vi "main(Test DQMH modules).vi"() -> ()   [LabVIEW 2018, in "Application.lvlib"] (continued)
        n1265 = Build Array("Apps.UI Update", "MEAS.AllRelaysOFF2", "Apps.WaitForEvent") -> (w2918:string[])
        n1266 = for {
          tunnel: [w2978] -> w2924 mode=indexing
          shift-right: [w2979] -> w2925
          shift-left: w2920 -> [w2977]
          tunnel: w2918 -> [w2976] mode=indexing
          n1267 = call "App enquece.vi"("Priority Enquece"=TRUE, "command"=w2976, "queue in"=w2977) -> ("error out"=w2978:errorcluster, "Queue out"=w2979:refnum<queue>)  [unwired: 7 in]
        }
        n1268 = call "FGV DRV stand.vi"() -> ("Sub-Test.DCV"=w2910:bool)  [unwired: 10 in, 1 out]
        n1269 = case shown="True" w2910 {
          tunnel: [w2965 w2975] -> w2926
          frame False {
            n1270 = Build Array("WaitFor", "MEAS.requestAC") -> (w2965:string[])
          }
          frame True {
            n1271 = Build Array("Test DRV 37", "Test DRV 38", "Test DRV 39", "Test DRV 40", "Test DRV 41", "Test DRV 42", "MEAS.requestAC") -> (w2975:string[])
          }
        }
        n1272 = Merge Errors(w2924) -> (w2917:errorcluster)
        n1273 = Reverse 1D Array(array=w2926) -> (reversed array=w2927:string[])
        n1274 = for {
          tunnel: w2927 -> [w2985] mode=indexing
          tunnel: [w2984] -> w2923 mode=indexing
          shift-right: [w2983] -> w2916
          shift-left: w2925 -> [w2986]
          tunnel: w2917 -> [w2982]
          n1275 = call "App enquece.vi"("Priority Enquece"=TRUE, "error in (no error)"=w2982, "command"=w2985, "queue in"=w2986) -> ("error out"=w2984:errorcluster, "Queue out"=w2983:refnum<queue>)  [unwired: 6 in]
        }
        n1276 = call "FGV DRV stand.vi"() -> ("Sub-Test.DCV"=w2909:bool)  [unwired: 10 in, 1 out]
        n1277 = Merge Errors(w2923) -> (w2922:errorcluster)
        n1278 = case shown="False" w2909 {
          tunnel: [w2938 w2954] -> w2921
          frame True {
            w2939 = T9 {"command"="", "data"=variant} ("element")
            n1279 = Initialize Array(TRUE, 6 ("dimension size")) -> (w2942:bool[])
            n1280 = To Variant(anything=T3."mux10_1_channel7" ("mux10_1(x6)_encode")) -> (Variant=w2951:variant)
            n1281 = To Variant(anything=T4."demux1_10_channel7" ("demux1_10(x6)_encode")) -> (Variant=w2947:variant)
            n1282 = To Variant(anything=w2942) -> (Variant=w2941:variant)
            n1283 = Bundle By Name(cluster=w2939, "command"="MEAS.mux10-1", "data"=w2951) -> (w2946:T9)
            n1284 = Bundle By Name(cluster=w2939, "command"="MEAS.demux1-10", "data"=w2947) -> (w2945:T9)
            n1285 = Bundle By Name(cluster=w2939, "command"="MEAS.eMIC", "data"=w2941) -> (w2940:T9)
            n1286 = Build Array(w2946, w2945, w2940) -> (w2938:T9[])
          }
          frame False {
            w2955 = T9 {"command"="", "data"=variant} ("element")
            n1287 = Initialize Array(TRUE, 6 ("dimension size")) -> (w2958:bool[])
            n1288 = To Variant(anything=T4."demux1_10_channel7" ("demux1_10(x6)_encode")) -> (Variant=w2962:variant)
            n1289 = To Variant(anything=w2958) -> (Variant=w2957:variant)
            n1290 = Bundle By Name(cluster=w2955, "command"="MEAS.demux1-10", "data"=w2962) -> (w2961:T9)
            n1291 = Bundle By Name(cluster=w2955, "command"="MEAS.eMIC", "data"=w2957) -> (w2956:T9)
            n1292 = Build Array(w2961, w2956) -> (w2954:T9[])
          }
        }
        n1293 = Reverse 1D Array(array=w2921) -> (reversed array=w2915:T9[])
        n1294 = for {
          tunnel: w2915 -> [w2997] mode=indexing
          tunnel: [w2994] -> w2928 mode=indexing
          tunnel: w2922 -> [w2993]
          tunnel: w2916 -> [w2991]
          n1295 = Unbundle By Name(w2997) -> ("command"=w2996:string, "data"=w2995:variant)
          n1296 = call "App enquece.vi"("Priority Enquece"=TRUE, "error in (no error)"=w2993, "command data"=w2995, "command"=w2996, "queue in"=w2991) -> ("error out"=w2994:errorcluster)  [unwired: 5 in, 1 out]
        }
        n1297 = Merge Errors(w2931, w2928) -> (w2932:errorcluster)
      }
      frame "Test Channel 8" {
        w2999 = T9 {"command"="", "data"=variant} ("element")
        w3037 = 8  # DUT channel (1-10)
        n1298 = disable-structure shown="LOGGING==TRUE" {
          disable-tunnel: w3032 -> [w3063 _]
          frame condition #0 (active) {
            n1299 = Empty String/Path?(string/path=w3063) -> (empty?=w3065:bool)
            n1300 = Select(t="Quece timeout", s=w3065, f=w3063) -> (s? t:f=w3062:string)
            n1301 = call "string log (SubVI).vi"("state Name"=w3062) -> ()  [unwired: 9 in, 2 out]
          }
          frame condition #1 {
          }
        }
        n1302 = Build Array("Apps.UI Update", "MEAS.AllRelaysOFF2", "Apps.WaitForEvent") -> (w3019:string[])
        n1303 = for {
          tunnel: [w3053] -> w3026 mode=indexing
          shift-right: [w3054] -> w3028
          shift-left: w3021 -> [w3052]
          tunnel: w3019 -> [w3051] mode=indexing
          n1304 = call "App enquece.vi"("Priority Enquece"=TRUE, "command"=w3051, "queue in"=w3052) -> ("error out"=w3053:errorcluster, "Queue out"=w3054:refnum<queue>)  [unwired: 7 in]
        }
        n1305 = call "FGV DRV stand.vi"() -> ("Sub-Test.DCV"=w3013:bool)  [unwired: 10 in, 1 out]
        n1306 = case shown="True" w3013 {
          tunnel: [w3040 w3050] -> w3029
          frame False {
            n1307 = Build Array("WaitFor", "MEAS.requestAC") -> (w3040:string[])
          }
          frame True {
            n1308 = Build Array("Test DRV 43", "Test DRV 44", "Test DRV 45", "Test DRV 46", "Test DRV 47", "Test DRV 48", "MEAS.requestAC") -> (w3050:string[])
          }
        }
        n1309 = Merge Errors(w3026) -> (w3018:errorcluster)
        n1310 = Reverse 1D Array(array=w3029) -> (reversed array=w3030:string[])
        n1311 = for {
          tunnel: w3030 -> [w3060] mode=indexing
          tunnel: [w3059] -> w3025 mode=indexing
          shift-right: [w3058] -> w3027
          shift-left: w3028 -> [w3061]
          tunnel: w3018 -> [w3057]
          n1312 = call "App enquece.vi"("Priority Enquece"=TRUE, "error in (no error)"=w3057, "command"=w3060, "queue in"=w3061) -> ("error out"=w3059:errorcluster, "Queue out"=w3058:refnum<queue>)  [unwired: 6 in]
        }
        n1313 = Merge Errors(w3025) -> (w3024:errorcluster)
        n1314 = Initialize Array(TRUE, 6 ("dimension size")) -> (w3002:bool[])
        n1315 = To Variant(anything=T3."mux10_1_channel8" ("mux10_1(x6)_encode")) -> (Variant=w3011:variant)
        n1316 = To Variant(anything=T4."demux1_10_channel8" ("demux1_10(x6)_encode")) -> (Variant=w3007:variant)
        n1317 = To Variant(anything=w3002) -> (Variant=w3001:variant)
        n1318 = Bundle By Name(cluster=w2999, "command"="MEAS.mux10-1", "data"=w3011) -> (w3006:T9)
        n1319 = Bundle By Name(cluster=w2999, "command"="MEAS.demux1-10", "data"=w3007) -> (w3005:T9)
        n1320 = Bundle By Name(cluster=w2999, "command"="MEAS.eMIC", "data"=w3001) -> (w3000:T9)
        n1321 = Build Array(w3006, w3005, w3000) -> (w3023:T9[])
        n1322 = Reverse 1D Array(array=w3023) -> (reversed array=w3022:T9[])
        n1323 = for {
          tunnel: w3022 -> [w3071] mode=indexing
          tunnel: [w3068] -> w3031 mode=indexing
          tunnel: w3024 -> [w3067]
          tunnel: w3027 -> [w3072]
          n1324 = Unbundle By Name(w3071) -> ("command"=w3070:string, "data"=w3069:variant)
          n1325 = call "App enquece.vi"("Priority Enquece"=TRUE, "error in (no error)"=w3067, "command data"=w3069, "command"=w3070, "queue in"=w3072) -> ("error out"=w3068:errorcluster)  [unwired: 5 in, 1 out]
        }
        n1326 = Merge Errors(w3034, w3031) -> (w3035:errorcluster)
      }
      frame "Test Channel 9" {
        w3074 = T9 {"command"="", "data"=variant} ("element")
        w3113 = 9  # DUT channel (1-10)
        n1327 = disable-structure shown="LOGGING==TRUE" {
          disable-tunnel: w3108 -> [w3138 _]
          frame condition #0 (active) {
            n1328 = Empty String/Path?(string/path=w3138) -> (empty?=w3140:bool)
            n1329 = Select(t="Quece timeout", s=w3140, f=w3138) -> (s? t:f=w3137:string)
            n1330 = call "string log (SubVI).vi"("state Name"=w3137) -> ()  [unwired: 9 in, 2 out]
          }
          frame condition #1 {
          }
        }
        n1331 = Build Array("Apps.UI Update", "MEAS.AllRelaysOFF2", "Apps.WaitForEvent") -> (w3094:string[])
        n1332 = for {
          tunnel: [w3128] -> w3102 mode=indexing
          shift-right: [w3129] -> w3104
          shift-left: w3097 -> [w3127]
          tunnel: w3094 -> [w3126] mode=indexing
          n1333 = call "App enquece.vi"("Priority Enquece"=TRUE, "command"=w3126, "queue in"=w3127) -> ("error out"=w3128:errorcluster, "Queue out"=w3129:refnum<queue>)  [unwired: 7 in]
        }
        n1334 = call "FGV DRV stand.vi"() -> ("Sub-Test.DCV"=w3088:bool)  [unwired: 10 in, 1 out]
        n1335 = Merge Errors(w3102) -> (w3093:errorcluster)
        n1336 = case shown="True" w3088 {
          tunnel: [w3115 w3125] -> w3105
          frame False {
            n1337 = Build Array("WaitFor", "MEAS.requestAC") -> (w3115:string[])
          }
          frame True {
            n1338 = Build Array("Test DRV 49", "Test DRV 50", "Test DRV 51", "Test DRV 52", "Test DRV 53", "Test DRV 54", "MEAS.requestAC") -> (w3125:string[])
          }
        }
        n1339 = Reverse 1D Array(array=w3105) -> (reversed array=w3106:string[])
        n1340 = for {
          tunnel: w3106 -> [w3135] mode=indexing
          tunnel: [w3134] -> w3101 mode=indexing
          shift-right: [w3133] -> w3103
          shift-left: w3104 -> [w3136]
          tunnel: w3093 -> [w3132]
          n1341 = call "App enquece.vi"("Priority Enquece"=TRUE, "error in (no error)"=w3132, "command"=w3135, "queue in"=w3136) -> ("error out"=w3134:errorcluster, "Queue out"=w3133:refnum<queue>)  [unwired: 6 in]
        }
        n1342 = Merge Errors(w3101) -> (w3100:errorcluster)
        n1343 = Initialize Array(TRUE, 6 ("dimension size")) -> (w3077:bool[])
        n1344 = To Variant(anything=T3."mux10_1_channel9" ("mux10_1(x6)_encode")) -> (Variant=w3086:variant)
        n1345 = To Variant(anything=T4."demux1_10_channel9" ("demux1_10(x6)_encode")) -> (Variant=w3082:variant)
        n1346 = To Variant(anything=w3077) -> (Variant=w3076:variant)
        n1347 = Bundle By Name(cluster=w3074, "command"="MEAS.mux10-1", "data"=w3086) -> (w3081:T9)
        n1348 = Bundle By Name(cluster=w3074, "command"="MEAS.demux1-10", "data"=w3082) -> (w3080:T9)
        n1349 = Bundle By Name(cluster=w3074, "command"="MEAS.eMIC", "data"=w3076) -> (w3075:T9)
        n1350 = Build Array(w3081, w3080, w3075) -> (w3099:T9[])
        n1351 = Reverse 1D Array(array=w3099) -> (reversed array=w3098:T9[])
        n1352 = for {
          tunnel: w3098 -> [w3146] mode=indexing
          tunnel: [w3143] -> w3107 mode=indexing
          tunnel: w3100 -> [w3142]
          tunnel: w3103 -> [w3147]
          n1353 = Unbundle By Name(w3146) -> ("command"=w3145:string, "data"=w3144:variant)
          n1354 = call "App enquece.vi"("Priority Enquece"=TRUE, "error in (no error)"=w3142, "command data"=w3144, "command"=w3145, "queue in"=w3147) -> ("error out"=w3143:errorcluster)  [unwired: 5 in, 1 out]
        }
        n1355 = Merge Errors(w3110, w3107) -> (w3111:errorcluster)
      }
      frame "Test Channel 10" {
        w3150 = T9 {"command"="", "data"=variant} ("element")
        w3187 = 10  # DUT channel (1-10)
        n1356 = disable-structure shown="LOGGING==TRUE" {
          disable-tunnel: w3183 -> [w3213 _]
          frame condition #0 (active) {
            n1357 = Empty String/Path?(string/path=w3213) -> (empty?=w3215:bool)
            n1358 = Select(t="Quece timeout", s=w3215, f=w3213) -> (s? t:f=w3212:string)
            n1359 = call "string log (SubVI).vi"("state Name"=w3212) -> ()  [unwired: 9 in, 2 out]
          }
          frame condition #1 {
          }
        }
        n1360 = Build Array("Apps.UI Update", "MEAS.AllRelaysOFF2", "Apps.WaitForEvent") -> (w3170:string[])
        n1361 = for {
          tunnel: [w3203] -> w3177 mode=indexing
          shift-right: [w3204] -> w3179
          shift-left: w3172 -> [w3202]
          tunnel: w3170 -> [w3201] mode=indexing
          n1362 = call "App enquece.vi"("Priority Enquece"=TRUE, "command"=w3201, "queue in"=w3202) -> ("error out"=w3203:errorcluster, "Queue out"=w3204:refnum<queue>)  [unwired: 7 in]
        }
        n1363 = call "FGV DRV stand.vi"() -> ("Sub-Test.DCV"=w3164:bool)  [unwired: 10 in, 1 out]
        n1364 = case shown="True" w3164 {
          tunnel: [w3190 w3200] -> w3180
          frame False {
            n1365 = Build Array("WaitFor", "MEAS.requestAC") -> (w3190:string[])
          }
          frame True {
            n1366 = Build Array("Test DRV 55", "Test DRV 56", "Test DRV 57", "Test DRV 58", "Test DRV 59", "Test DRV 60", "MEAS.requestAC") -> (w3200:string[])
          }
        }
        n1367 = Merge Errors(w3177) -> (w3169:errorcluster)
        n1368 = Reverse 1D Array(array=w3180) -> (reversed array=w3181:string[])
        n1369 = for {
          tunnel: w3181 -> [w3210] mode=indexing
          tunnel: [w3209] -> w3176 mode=indexing
          shift-right: [w3208] -> w3178
          shift-left: w3179 -> [w3211]
          tunnel: w3169 -> [w3207]
          n1370 = call "App enquece.vi"("Priority Enquece"=TRUE, "error in (no error)"=w3207, "command"=w3210, "queue in"=w3211) -> ("error out"=w3209:errorcluster, "Queue out"=w3208:refnum<queue>)  [unwired: 6 in]
        }
        n1371 = Merge Errors(w3176) -> (w3175:errorcluster)
        n1372 = Initialize Array(TRUE, 6 ("dimension size")) -> (w3148:bool[])
        n1373 = To Variant(anything=T3."mux10_1_channel10" ("mux10_1(x6)_encode")) -> (Variant=w3161:variant)
        n1374 = To Variant(anything=T4."demux1_10_channel10" ("demux1_10(x6)_encode")) -> (Variant=w3157:variant)
        n1375 = To Variant(anything=w3148) -> (Variant=w3153:variant)
        n1376 = Bundle By Name(cluster=w3150, "command"="MEAS.mux10-1", "data"=w3161) -> (w3156:T9)
        n1377 = Bundle By Name(cluster=w3150, "command"="MEAS.demux1-10", "data"=w3157) -> (w3155:T9)
        n1378 = Bundle By Name(cluster=w3150, "command"="MEAS.eMIC", "data"=w3153) -> (w3152:T9)
        n1379 = Build Array(w3156, w3155, w3152) -> (w3174:T9[])
        n1380 = Reverse 1D Array(array=w3174) -> (reversed array=w3173:T9[])
        n1381 = for {
          tunnel: w3173 -> [w3221] mode=indexing
          tunnel: [w3218] -> w3182 mode=indexing
          tunnel: w3175 -> [w3217]
          tunnel: w3178 -> [w3222]
          n1382 = Unbundle By Name(w3221) -> ("command"=w3220:string, "data"=w3219:variant)
          n1383 = call "App enquece.vi"("Priority Enquece"=TRUE, "error in (no error)"=w3217, "command data"=w3219, "command"=w3220, "queue in"=w3222) -> ("error out"=w3218:errorcluster)  [unwired: 5 in, 1 out]
        }
        n1384 = Merge Errors(w3185, w3182) -> (w3163:errorcluster)
      }
      frame "Test Channel 10A" {
        w3229 = T9 {"command"="", "data"=variant} ("element")
        w3250 = T9 {"command"="", "data"=variant} ("element")
        w3271 = 10  # DUT channel (1-10)
        n1385 = disable-structure shown="LOGGING==TRUE" {
          disable-tunnel: w3266 -> [w3295 _]
          frame condition #0 (active) {
            n1386 = Empty String/Path?(string/path=w3295) -> (empty?=w3297:bool)
            n1387 = Select(t="Quece timeout", s=w3297, f=w3295) -> (s? t:f=w3294:string)
            n1388 = call "string log (SubVI).vi"("state Name"=w3294) -> ()  [unwired: 9 in, 2 out]
          }
          frame condition #1 {
          }
        }
        n1389 = Bundle By Name(cluster=w3250, "command"="Apps.UI Update", "data"="A") -> (w3249:T9)
        n1390 = Bundle By Name(cluster=w3250, "command"="MEAS.AllRelaysOFF2") -> (w3248:T9)
        n1391 = Bundle By Name(cluster=w3250, "command"="Apps.WaitForEvent") -> (w3247:T9)
        n1392 = Build Array(w3249, w3248, w3247) -> (w3255:T9[])
        n1393 = call "FGV DRV stand.vi"() -> ("Sub-Test.DCV"=w3243:bool)  [unwired: 10 in, 1 out]
        n1394 = for {
          tunnel: [w3285] -> w3261 mode=indexing
          shift-right: [w3286] -> w3263
          shift-left: w3256 -> [w3284]
          tunnel: w3255 -> [w3283] mode=indexing
          n1395 = Unbundle By Name(w3283) -> ("command"=w3282:string, "data"=w3281:variant)
          n1396 = call "App enquece.vi"("Priority Enquece"=TRUE, "command data"=w3281, "command"=w3282, "queue in"=w3284) -> ("error out"=w3285:errorcluster, "Queue out"=w3286:refnum<queue>)  [unwired: 6 in]
        }
        n1397 = case shown="True" w3243 {
          tunnel: [w3274 w3280] -> w3264
          frame False {
            n1398 = Build Array("WaitFor", "MEAS.requestAC") -> (w3274:string[])
          }
          frame True {
            n1399 = Build Array("Test DRV 55", "WaitForA", "MEAS.requestAC") -> (w3280:string[])
          }
        }
        n1400 = Merge Errors(w3261) -> (w3254:errorcluster)
        n1401 = Reverse 1D Array(array=w3264) -> (reversed array=w3242:string[])
        n1402 = for {
          tunnel: w3242 -> [w3292] mode=indexing
          tunnel: [w3291] -> w3260 mode=indexing
          shift-right: [w3290] -> w3262
          shift-left: w3263 -> [w3293]
          tunnel: w3254 -> [w3289]
          n1403 = call "App enquece.vi"("Priority Enquece"=TRUE, "error in (no error)"=w3289, "command"=w3292, "queue in"=w3293) -> ("error out"=w3291:errorcluster, "Queue out"=w3290:refnum<queue>)  [unwired: 6 in]
        }
        n1404 = Merge Errors(w3260) -> (w3259:errorcluster)
        n1405 = Initialize Array(FALSE ("element"), 6 ("dimension size")) -> (w3225:bool[])
        n1406 = Initialize Array(TRUE, 1 ("dimension size")) -> (w3224:bool[])
        n1407 = Replace Array Subset(array=w3225, new element=w3224) -> (w3223:bool[])  [unwired: 1 in]
        n1408 = To Variant(anything=T3."mux10_1_channel10" ("mux10_1(x6)_encode")) -> (Variant=w3240:variant)
        n1409 = To Variant(anything=T4."demux1_10_channel10" ("demux1_10(x6)_encode")) -> (Variant=w3236:variant)
        n1410 = To Variant(anything=w3223) -> (Variant=w3232:variant)
        n1411 = Bundle By Name(cluster=w3229, "command"="MEAS.mux10-1", "data"=w3240) -> (w3235:T9)
        n1412 = Bundle By Name(cluster=w3229, "command"="MEAS.demux1-10", "data"=w3236) -> (w3234:T9)
        n1413 = Bundle By Name(cluster=w3229, "command"="MEAS.eMIC", "data"=w3232) -> (w3231:T9)
        n1414 = Build Array(w3235, w3234, w3231) -> (w3258:T9[])
        n1415 = Reverse 1D Array(array=w3258) -> (reversed array=w3257:T9[])
        n1416 = for {
          tunnel: w3257 -> [w3303] mode=indexing
          tunnel: [w3300] -> w3265 mode=indexing
          tunnel: w3259 -> [w3299]
          tunnel: w3262 -> [w3304]
          n1417 = Unbundle By Name(w3303) -> ("command"=w3302:string, "data"=w3301:variant)
          n1418 = call "App enquece.vi"("Priority Enquece"=TRUE, "error in (no error)"=w3299, "command data"=w3301, "command"=w3302, "queue in"=w3304) -> ("error out"=w3300:errorcluster)  [unwired: 5 in, 1 out]
        }
        n1419 = Merge Errors(w3268, w3265) -> (w3269:errorcluster)
      }
      frame "Test Channel 1A" {
        w3311 = T9 {"command"="", "data"=variant} ("element")
        w3332 = T9 {"command"="", "data"=variant} ("element")
        w3353 = 1  # DUT channel (1-10)
        n1420 = disable-structure shown="LOGGING==TRUE" {
          disable-tunnel: w3348 -> [w3377 _]
          frame condition #0 (active) {
            n1421 = Empty String/Path?(string/path=w3377) -> (empty?=w3379:bool)
            n1422 = Select(t="Quece timeout", s=w3379, f=w3377) -> (s? t:f=w3376:string)
            n1423 = call "string log (SubVI).vi"("state Name"=w3376) -> ()  [unwired: 9 in, 2 out]
          }
          frame condition #1 {
          }
        }
        n1424 = Bundle By Name(cluster=w3332, "command"="Apps.UI Update", "data"="A") -> (w3331:T9)
        n1425 = Bundle By Name(cluster=w3332, "command"="MEAS.AllRelaysOFF2") -> (w3330:T9)
        n1426 = Bundle By Name(cluster=w3332, "command"="Apps.WaitForEvent") -> (w3329:T9)
        n1427 = Build Array(w3331, w3330, w3329) -> (w3337:T9[])
        n1428 = for {
          tunnel: [w3367] -> w3343 mode=indexing
          shift-right: [w3368] -> w3345
          shift-left: w3338 -> [w3366]
          tunnel: w3337 -> [w3365] mode=indexing
          n1429 = Unbundle By Name(w3365) -> ("command"=w3364:string, "data"=w3363:variant)
          n1430 = call "App enquece.vi"("Priority Enquece"=TRUE, "command data"=w3363, "command"=w3364, "queue in"=w3366) -> ("error out"=w3367:errorcluster, "Queue out"=w3368:refnum<queue>)  [unwired: 6 in]
        }
        n1431 = call "FGV DRV stand.vi"() -> ("Sub-Test.DCV"=w3325:bool)  [unwired: 10 in, 1 out]
        n1432 = case shown="True" w3325 {
          tunnel: [w3356 w3362] -> w3346
          frame False {
            n1433 = Build Array("WaitFor", "MEAS.requestAC") -> (w3356:string[])
          }
          frame True {
            n1434 = Build Array("Test DRV 1", "WaitForA", "MEAS.requestAC") -> (w3362:string[])
          }
        }
        n1435 = Merge Errors(w3343) -> (w3336:errorcluster)
        n1436 = Reverse 1D Array(array=w3346) -> (reversed array=w3324:string[])
        n1437 = for {
          tunnel: w3324 -> [w3374] mode=indexing
          tunnel: [w3373] -> w3342 mode=indexing
          shift-right: [w3372] -> w3344
          shift-left: w3345 -> [w3375]
          tunnel: w3336 -> [w3371]
          n1438 = call "App enquece.vi"("Priority Enquece"=TRUE, "error in (no error)"=w3371, "command"=w3374, "queue in"=w3375) -> ("error out"=w3373:errorcluster, "Queue out"=w3372:refnum<queue>)  [unwired: 6 in]
        }
        n1439 = Merge Errors(w3342) -> (w3341:errorcluster)
        n1440 = Initialize Array(FALSE ("element"), 6 ("dimension size")) -> (w3307:bool[])
        n1441 = Initialize Array(TRUE, 1 ("dimension size")) -> (w3306:bool[])
        n1442 = Replace Array Subset(array=w3307, new element=w3306) -> (w3305:bool[])  [unwired: 1 in]
        n1443 = To Variant(anything=T3."mux10_1_channel1" ("mux10_1(x6)_encode")) -> (Variant=w3322:variant)
        n1444 = To Variant(anything=T4."demux1_10_channel1" ("demux1_10(x6)_encode")) -> (Variant=w3318:variant)
        n1445 = To Variant(anything=w3305) -> (Variant=w3314:variant)
        n1446 = Bundle By Name(cluster=w3311, "command"="MEAS.mux10-1", "data"=w3322) -> (w3317:T9)
        n1447 = Bundle By Name(cluster=w3311, "command"="MEAS.demux1-10", "data"=w3318) -> (w3316:T9)
        n1448 = Bundle By Name(cluster=w3311, "command"="MEAS.eMIC", "data"=w3314) -> (w3313:T9)
        n1449 = Build Array(w3317, w3316, w3313) -> (w3340:T9[])
        n1450 = Reverse 1D Array(array=w3340) -> (reversed array=w3339:T9[])
        n1451 = for {
          tunnel: w3339 -> [w3385] mode=indexing
          tunnel: [w3382] -> w3347 mode=indexing
          tunnel: w3341 -> [w3381]
          tunnel: w3344 -> [w3386]
          n1452 = Unbundle By Name(w3385) -> ("command"=w3384:string, "data"=w3383:variant)
          n1453 = call "App enquece.vi"("Priority Enquece"=TRUE, "error in (no error)"=w3381, "command data"=w3383, "command"=w3384, "queue in"=w3386) -> ("error out"=w3382:errorcluster)  [unwired: 5 in, 1 out]
        }
        n1454 = Merge Errors(w3350, w3347) -> (w3351:errorcluster)
      }
      frame "Test Channel 2A" {
        w3393 = T9 {"command"="", "data"=variant} ("element")
        w3414 = T9 {"command"="", "data"=variant} ("element")
        w3435 = 2  # DUT channel (1-10)
        n1455 = disable-structure shown="LOGGING==TRUE" {
          disable-tunnel: w3430 -> [w3459 _]
          frame condition #0 (active) {
            n1456 = Empty String/Path?(string/path=w3459) -> (empty?=w3461:bool)
            n1457 = Select(t="Quece timeout", s=w3461, f=w3459) -> (s? t:f=w3458:string)
            n1458 = call "string log (SubVI).vi"("state Name"=w3458) -> ()  [unwired: 9 in, 2 out]
          }
          frame condition #1 {
          }
        }
        n1459 = Bundle By Name(cluster=w3414, "command"="Apps.UI Update", "data"="A") -> (w3413:T9)
        n1460 = Bundle By Name(cluster=w3414, "command"="MEAS.AllRelaysOFF2") -> (w3412:T9)
        n1461 = Bundle By Name(cluster=w3414, "command"="Apps.WaitForEvent") -> (w3411:T9)
        n1462 = Build Array(w3413, w3412, w3411) -> (w3419:T9[])
        n1463 = for {
          tunnel: [w3449] -> w3425 mode=indexing
          shift-right: [w3450] -> w3427
          shift-left: w3420 -> [w3448]
          tunnel: w3419 -> [w3447] mode=indexing
          n1464 = Unbundle By Name(w3447) -> ("command"=w3446:string, "data"=w3445:variant)
          n1465 = call "App enquece.vi"("Priority Enquece"=TRUE, "command data"=w3445, "command"=w3446, "queue in"=w3448) -> ("error out"=w3449:errorcluster, "Queue out"=w3450:refnum<queue>)  [unwired: 6 in]
        }
        n1466 = call "FGV DRV stand.vi"() -> ("Sub-Test.DCV"=w3407:bool)  [unwired: 10 in, 1 out]
        n1467 = case shown="True" w3407 {
          tunnel: [w3438 w3444] -> w3428
          frame False {
            n1468 = Build Array("WaitFor", "MEAS.requestAC") -> (w3438:string[])
          }
          frame True {
            n1469 = Build Array("Test DRV 7", "WaitForA", "MEAS.requestAC") -> (w3444:string[])
          }
        }
        n1470 = Merge Errors(w3425) -> (w3418:errorcluster)
        n1471 = Reverse 1D Array(array=w3428) -> (reversed array=w3406:string[])
        n1472 = for {
          tunnel: w3406 -> [w3456] mode=indexing
          tunnel: [w3455] -> w3424 mode=indexing
          shift-right: [w3454] -> w3426
          shift-left: w3427 -> [w3457]
          tunnel: w3418 -> [w3453]
          n1473 = call "App enquece.vi"("Priority Enquece"=TRUE, "error in (no error)"=w3453, "command"=w3456, "queue in"=w3457) -> ("error out"=w3455:errorcluster, "Queue out"=w3454:refnum<queue>)  [unwired: 6 in]
        }
        n1474 = Initialize Array(FALSE ("element"), 6 ("dimension size")) -> (w3389:bool[])
        n1475 = Merge Errors(w3424) -> (w3423:errorcluster)
        n1476 = Initialize Array(TRUE, 1 ("dimension size")) -> (w3388:bool[])
        n1477 = Replace Array Subset(array=w3389, new element=w3388) -> (w3387:bool[])  [unwired: 1 in]
        n1478 = To Variant(anything=T3."mux10_1_channel2" ("mux10_1(x6)_encode")) -> (Variant=w3404:variant)
        n1479 = To Variant(anything=T4."demux1_10_channel2" ("demux1_10(x6)_encode")) -> (Variant=w3400:variant)
        n1480 = To Variant(anything=w3387) -> (Variant=w3396:variant)
        n1481 = Bundle By Name(cluster=w3393, "command"="MEAS.mux10-1", "data"=w3404) -> (w3399:T9)
        n1482 = Bundle By Name(cluster=w3393, "command"="MEAS.demux1-10", "data"=w3400) -> (w3398:T9)
        n1483 = Bundle By Name(cluster=w3393, "command"="MEAS.eMIC", "data"=w3396) -> (w3395:T9)
        n1484 = Build Array(w3399, w3398, w3395) -> (w3422:T9[])
        n1485 = Reverse 1D Array(array=w3422) -> (reversed array=w3421:T9[])
        n1486 = for {
          tunnel: w3421 -> [w3467] mode=indexing
          tunnel: [w3464] -> w3429 mode=indexing
          tunnel: w3423 -> [w3463]
          tunnel: w3426 -> [w3468]
          n1487 = Unbundle By Name(w3467) -> ("command"=w3466:string, "data"=w3465:variant)
          n1488 = call "App enquece.vi"("Priority Enquece"=TRUE, "error in (no error)"=w3463, "command data"=w3465, "command"=w3466, "queue in"=w3468) -> ("error out"=w3464:errorcluster)  [unwired: 5 in, 1 out]
        }
        n1489 = Merge Errors(w3432, w3429) -> (w3433:errorcluster)
      }
      frame "Test Channel 3A" {
        w3475 = T9 {"command"="", "data"=variant} ("element")
        w3496 = T9 {"command"="", "data"=variant} ("element")
        w3517 = 3  # DUT channel (1-10)
        n1490 = disable-structure shown="LOGGING==TRUE" {
          disable-tunnel: w3512 -> [w3541 _]
          frame condition #0 (active) {
            n1491 = Empty String/Path?(string/path=w3541) -> (empty?=w3543:bool)
            n1492 = Select(t="Quece timeout", s=w3543, f=w3541) -> (s? t:f=w3540:string)
            n1493 = call "string log (SubVI).vi"("state Name"=w3540) -> ()  [unwired: 9 in, 2 out]
          }
          frame condition #1 {
          }
        }
        n1494 = Bundle By Name(cluster=w3496, "command"="Apps.UI Update", "data"="A") -> (w3495:T9)
        n1495 = Bundle By Name(cluster=w3496, "command"="MEAS.AllRelaysOFF2") -> (w3494:T9)
        n1496 = Bundle By Name(cluster=w3496, "command"="Apps.WaitForEvent") -> (w3493:T9)
        n1497 = Build Array(w3495, w3494, w3493) -> (w3501:T9[])
        n1498 = for {
          tunnel: [w3531] -> w3507 mode=indexing
          shift-right: [w3532] -> w3509
          shift-left: w3502 -> [w3530]
          tunnel: w3501 -> [w3529] mode=indexing
          n1499 = Unbundle By Name(w3529) -> ("command"=w3528:string, "data"=w3527:variant)
          n1500 = call "App enquece.vi"("Priority Enquece"=TRUE, "command data"=w3527, "command"=w3528, "queue in"=w3530) -> ("error out"=w3531:errorcluster, "Queue out"=w3532:refnum<queue>)  [unwired: 6 in]
        }
        n1501 = call "FGV DRV stand.vi"() -> ("Sub-Test.DCV"=w3489:bool)  [unwired: 10 in, 1 out]
        n1502 = case shown="True" w3489 {
          tunnel: [w3520 w3526] -> w3510
          frame False {
            n1503 = Build Array("WaitFor", "MEAS.requestAC") -> (w3520:string[])
          }
          frame True {
            n1504 = Build Array("Test DRV 13", "WaitForA", "MEAS.requestAC") -> (w3526:string[])
          }
        }
        n1505 = Merge Errors(w3507) -> (w3500:errorcluster)
        n1506 = Reverse 1D Array(array=w3510) -> (reversed array=w3488:string[])
        n1507 = for {
          tunnel: w3488 -> [w3538] mode=indexing
          tunnel: [w3537] -> w3506 mode=indexing
          shift-right: [w3536] -> w3508
          shift-left: w3509 -> [w3539]
          tunnel: w3500 -> [w3535]
          n1508 = call "App enquece.vi"("Priority Enquece"=TRUE, "error in (no error)"=w3535, "command"=w3538, "queue in"=w3539) -> ("error out"=w3537:errorcluster, "Queue out"=w3536:refnum<queue>)  [unwired: 6 in]
        }
        n1509 = Initialize Array(FALSE ("element"), 6 ("dimension size")) -> (w3471:bool[])
        n1510 = Initialize Array(TRUE, 1 ("dimension size")) -> (w3470:bool[])
        n1511 = Merge Errors(w3506) -> (w3505:errorcluster)
        n1512 = Replace Array Subset(array=w3471, new element=w3470) -> (w3469:bool[])  [unwired: 1 in]
        n1513 = To Variant(anything=T3."mux10_1_channel3" ("mux10_1(x6)_encode")) -> (Variant=w3486:variant)
        n1514 = To Variant(anything=T4."demux1_10_channel3" ("demux1_10(x6)_encode")) -> (Variant=w3482:variant)
        n1515 = To Variant(anything=w3469) -> (Variant=w3478:variant)
        n1516 = Bundle By Name(cluster=w3475, "command"="MEAS.mux10-1", "data"=w3486) -> (w3481:T9)
        n1517 = Bundle By Name(cluster=w3475, "command"="MEAS.demux1-10", "data"=w3482) -> (w3480:T9)
        n1518 = Bundle By Name(cluster=w3475, "command"="MEAS.eMIC", "data"=w3478) -> (w3477:T9)
        n1519 = Build Array(w3481, w3480, w3477) -> (w3504:T9[])
        n1520 = Reverse 1D Array(array=w3504) -> (reversed array=w3503:T9[])
        n1521 = for {
          tunnel: w3503 -> [w3549] mode=indexing
          tunnel: [w3546] -> w3511 mode=indexing
          tunnel: w3505 -> [w3545]
          tunnel: w3508 -> [w3550]
          n1522 = Unbundle By Name(w3549) -> ("command"=w3548:string, "data"=w3547:variant)
          n1523 = call "App enquece.vi"("Priority Enquece"=TRUE, "error in (no error)"=w3545, "command data"=w3547, "command"=w3548, "queue in"=w3550) -> ("error out"=w3546:errorcluster)  [unwired: 5 in, 1 out]
        }
        n1524 = Merge Errors(w3514, w3511) -> (w3515:errorcluster)
      }
      frame "Test Channel 4A" {
        w3557 = T9 {"command"="", "data"=variant} ("element")
        w3578 = T9 {"command"="", "data"=variant} ("element")
        w3599 = 4  # DUT channel (1-10)
        n1525 = disable-structure shown="LOGGING==TRUE" {
          disable-tunnel: w3594 -> [w3623 _]
          frame condition #0 (active) {
            n1526 = Empty String/Path?(string/path=w3623) -> (empty?=w3625:bool)
            n1527 = Select(t="Quece timeout", s=w3625, f=w3623) -> (s? t:f=w3622:string)
            n1528 = call "string log (SubVI).vi"("state Name"=w3622) -> ()  [unwired: 9 in, 2 out]
          }
          frame condition #1 {
          }
        }
        n1529 = Bundle By Name(cluster=w3578, "command"="Apps.UI Update", "data"="A") -> (w3577:T9)
        n1530 = Bundle By Name(cluster=w3578, "command"="MEAS.AllRelaysOFF2") -> (w3576:T9)
        n1531 = Bundle By Name(cluster=w3578, "command"="Apps.WaitForEvent") -> (w3575:T9)
        n1532 = Build Array(w3577, w3576, w3575) -> (w3583:T9[])
        n1533 = for {
          tunnel: [w3613] -> w3589 mode=indexing
          shift-right: [w3614] -> w3591
          shift-left: w3584 -> [w3612]
          tunnel: w3583 -> [w3611] mode=indexing
          n1534 = Unbundle By Name(w3611) -> ("command"=w3610:string, "data"=w3609:variant)
          n1535 = call "App enquece.vi"("Priority Enquece"=TRUE, "command data"=w3609, "command"=w3610, "queue in"=w3612) -> ("error out"=w3613:errorcluster, "Queue out"=w3614:refnum<queue>)  [unwired: 6 in]
        }
        n1536 = call "FGV DRV stand.vi"() -> ("Sub-Test.DCV"=w3571:bool)  [unwired: 10 in, 1 out]
        n1537 = case shown="True" w3571 {
          tunnel: [w3602 w3608] -> w3592
          frame False {
            n1538 = Build Array("WaitFor", "MEAS.requestAC") -> (w3602:string[])
          }
          frame True {
            n1539 = Build Array("Test DRV 19", "WaitForA", "MEAS.requestAC") -> (w3608:string[])
          }
        }
        n1540 = Merge Errors(w3589) -> (w3582:errorcluster)
        n1541 = Reverse 1D Array(array=w3592) -> (reversed array=w3570:string[])
        n1542 = for {
          tunnel: w3570 -> [w3620] mode=indexing
          tunnel: [w3619] -> w3588 mode=indexing
          shift-right: [w3618] -> w3590
          shift-left: w3591 -> [w3621]
          tunnel: w3582 -> [w3617]
          n1543 = call "App enquece.vi"("Priority Enquece"=TRUE, "error in (no error)"=w3617, "command"=w3620, "queue in"=w3621) -> ("error out"=w3619:errorcluster, "Queue out"=w3618:refnum<queue>)  [unwired: 6 in]
        }
        n1544 = Initialize Array(FALSE ("element"), 6 ("dimension size")) -> (w3553:bool[])
        n1545 = Initialize Array(TRUE, 1 ("dimension size")) -> (w3552:bool[])
        n1546 = Merge Errors(w3588) -> (w3587:errorcluster)
        n1547 = Replace Array Subset(array=w3553, new element=w3552) -> (w3551:bool[])  [unwired: 1 in]
        n1548 = To Variant(anything=T3."mux10_1_channel4" ("mux10_1(x6)_encode")) -> (Variant=w3568:variant)
        n1549 = To Variant(anything=T4."demux1_10_channel4" ("demux1_10(x6)_encode")) -> (Variant=w3564:variant)
        n1550 = To Variant(anything=w3551) -> (Variant=w3560:variant)
        n1551 = Bundle By Name(cluster=w3557, "command"="MEAS.mux10-1", "data"=w3568) -> (w3563:T9)
        n1552 = Bundle By Name(cluster=w3557, "command"="MEAS.demux1-10", "data"=w3564) -> (w3562:T9)
        n1553 = Bundle By Name(cluster=w3557, "command"="MEAS.eMIC", "data"=w3560) -> (w3559:T9)
        n1554 = Build Array(w3563, w3562, w3559) -> (w3586:T9[])
        n1555 = Reverse 1D Array(array=w3586) -> (reversed array=w3585:T9[])
        n1556 = for {
          tunnel: w3585 -> [w3631] mode=indexing
          tunnel: [w3628] -> w3593 mode=indexing
          tunnel: w3587 -> [w3627]
          tunnel: w3590 -> [w3632]
          n1557 = Unbundle By Name(w3631) -> ("command"=w3630:string, "data"=w3629:variant)
          n1558 = call "App enquece.vi"("Priority Enquece"=TRUE, "error in (no error)"=w3627, "command data"=w3629, "command"=w3630, "queue in"=w3632) -> ("error out"=w3628:errorcluster)  [unwired: 5 in, 1 out]
        }
        n1559 = Merge Errors(w3596, w3593) -> (w3597:errorcluster)
      }
      frame "Test Channel 5A" {
        w3639 = T9 {"command"="", "data"=variant} ("element")
        w3660 = T9 {"command"="", "data"=variant} ("element")
        w3681 = 5  # DUT channel (1-10)
        n1560 = disable-structure shown="LOGGING==TRUE" {
          disable-tunnel: w3676 -> [w3705 _]
          frame condition #0 (active) {
            n1561 = Empty String/Path?(string/path=w3705) -> (empty?=w3707:bool)
            n1562 = Select(t="Quece timeout", s=w3707, f=w3705) -> (s? t:f=w3704:string)
            n1563 = call "string log (SubVI).vi"("state Name"=w3704) -> ()  [unwired: 9 in, 2 out]
          }
          frame condition #1 {
          }
        }
        n1564 = Bundle By Name(cluster=w3660, "command"="Apps.UI Update", "data"="A") -> (w3659:T9)
        n1565 = Bundle By Name(cluster=w3660, "command"="MEAS.AllRelaysOFF2") -> (w3658:T9)
        n1566 = Bundle By Name(cluster=w3660, "command"="Apps.WaitForEvent") -> (w3657:T9)
        n1567 = Build Array(w3659, w3658, w3657) -> (w3665:T9[])
        n1568 = for {
          tunnel: [w3695] -> w3671 mode=indexing
          shift-right: [w3696] -> w3673
          shift-left: w3666 -> [w3694]
          tunnel: w3665 -> [w3693] mode=indexing
          n1569 = Unbundle By Name(w3693) -> ("command"=w3692:string, "data"=w3691:variant)
          n1570 = call "App enquece.vi"("Priority Enquece"=TRUE, "command data"=w3691, "command"=w3692, "queue in"=w3694) -> ("error out"=w3695:errorcluster, "Queue out"=w3696:refnum<queue>)  [unwired: 6 in]
        }
        n1571 = call "FGV DRV stand.vi"() -> ("Sub-Test.DCV"=w3653:bool)  [unwired: 10 in, 1 out]
        n1572 = case shown="True" w3653 {
          tunnel: [w3684 w3690] -> w3674
          frame False {
            n1573 = Build Array("WaitFor", "MEAS.requestAC") -> (w3684:string[])
          }
          frame True {
            n1574 = Build Array("Test DRV 25", "WaitForA", "MEAS.requestAC") -> (w3690:string[])
          }
        }
        n1575 = Merge Errors(w3671) -> (w3664:errorcluster)
        n1576 = Reverse 1D Array(array=w3674) -> (reversed array=w3652:string[])
        n1577 = for {
          tunnel: w3652 -> [w3702] mode=indexing
          tunnel: [w3701] -> w3670 mode=indexing
          shift-right: [w3700] -> w3672
          shift-left: w3673 -> [w3703]
          tunnel: w3664 -> [w3699]
          n1578 = call "App enquece.vi"("Priority Enquece"=TRUE, "error in (no error)"=w3699, "command"=w3702, "queue in"=w3703) -> ("error out"=w3701:errorcluster, "Queue out"=w3700:refnum<queue>)  [unwired: 6 in]
        }
        n1579 = Initialize Array(FALSE ("element"), 6 ("dimension size")) -> (w3635:bool[])
        n1580 = Initialize Array(TRUE, 1 ("dimension size")) -> (w3634:bool[])
        n1581 = Replace Array Subset(array=w3635, new element=w3634) -> (w3633:bool[])  [unwired: 1 in]
        n1582 = Merge Errors(w3670) -> (w3669:errorcluster)
        n1583 = To Variant(anything=T3."mux10_1_channel5" ("mux10_1(x6)_encode")) -> (Variant=w3650:variant)
        n1584 = To Variant(anything=T4."demux1_10_channel5" ("demux1_10(x6)_encode")) -> (Variant=w3646:variant)
        n1585 = To Variant(anything=w3633) -> (Variant=w3642:variant)
        n1586 = Bundle By Name(cluster=w3639, "command"="MEAS.mux10-1", "data"=w3650) -> (w3645:T9)
        n1587 = Bundle By Name(cluster=w3639, "command"="MEAS.demux1-10", "data"=w3646) -> (w3644:T9)
        n1588 = Bundle By Name(cluster=w3639, "command"="MEAS.eMIC", "data"=w3642) -> (w3641:T9)
        n1589 = Build Array(w3645, w3644, w3641) -> (w3668:T9[])
        n1590 = Reverse 1D Array(array=w3668) -> (reversed array=w3667:T9[])
        n1591 = for {
          tunnel: w3667 -> [w3713] mode=indexing
          tunnel: [w3710] -> w3675 mode=indexing
          tunnel: w3669 -> [w3709]
          tunnel: w3672 -> [w3714]
          n1592 = Unbundle By Name(w3713) -> ("command"=w3712:string, "data"=w3711:variant)
          n1593 = call "App enquece.vi"("Priority Enquece"=TRUE, "error in (no error)"=w3709, "command data"=w3711, "command"=w3712, "queue in"=w3714) -> ("error out"=w3710:errorcluster)  [unwired: 5 in, 1 out]
        }
        n1594 = Merge Errors(w3678, w3675) -> (w3679:errorcluster)
      }
      frame "Test Channel 6A" {
        w3721 = T9 {"command"="", "data"=variant} ("element")
        w3742 = T9 {"command"="", "data"=variant} ("element")
        w3763 = 6  # DUT channel (1-10)
        n1595 = disable-structure shown="LOGGING==TRUE" {
          disable-tunnel: w3758 -> [w3787 _]
          frame condition #0 (active) {
            n1596 = Empty String/Path?(string/path=w3787) -> (empty?=w3789:bool)
            n1597 = Select(t="Quece timeout", s=w3789, f=w3787) -> (s? t:f=w3786:string)
            n1598 = call "string log (SubVI).vi"("state Name"=w3786) -> ()  [unwired: 9 in, 2 out]
          }
          frame condition #1 {
          }
        }
        n1599 = Bundle By Name(cluster=w3742, "command"="Apps.UI Update", "data"="A") -> (w3741:T9)
        n1600 = Bundle By Name(cluster=w3742, "command"="MEAS.AllRelaysOFF2") -> (w3740:T9)
        n1601 = Bundle By Name(cluster=w3742, "command"="Apps.WaitForEvent") -> (w3739:T9)
        n1602 = Build Array(w3741, w3740, w3739) -> (w3747:T9[])
        n1603 = for {
          tunnel: [w3777] -> w3753 mode=indexing
          shift-right: [w3778] -> w3755
          shift-left: w3748 -> [w3776]
          tunnel: w3747 -> [w3775] mode=indexing
          n1604 = Unbundle By Name(w3775) -> ("command"=w3774:string, "data"=w3773:variant)
          n1605 = call "App enquece.vi"("Priority Enquece"=TRUE, "command data"=w3773, "command"=w3774, "queue in"=w3776) -> ("error out"=w3777:errorcluster, "Queue out"=w3778:refnum<queue>)  [unwired: 6 in]
        }
        n1606 = call "FGV DRV stand.vi"() -> ("Sub-Test.DCV"=w3735:bool)  [unwired: 10 in, 1 out]
        n1607 = case shown="True" w3735 {
          tunnel: [w3766 w3772] -> w3756
          frame False {
            n1608 = Build Array("WaitFor", "MEAS.requestAC") -> (w3766:string[])
          }
          frame True {
            n1609 = Build Array("Test DRV 31", "WaitForA", "MEAS.requestAC") -> (w3772:string[])
          }
        }
        n1610 = Merge Errors(w3753) -> (w3746:errorcluster)
        n1611 = Reverse 1D Array(array=w3756) -> (reversed array=w3734:string[])
        n1612 = for {
          tunnel: w3734 -> [w3784] mode=indexing
          tunnel: [w3783] -> w3752 mode=indexing
          shift-right: [w3782] -> w3754
          shift-left: w3755 -> [w3785]
          tunnel: w3746 -> [w3781]
          n1613 = call "App enquece.vi"("Priority Enquece"=TRUE, "error in (no error)"=w3781, "command"=w3784, "queue in"=w3785) -> ("error out"=w3783:errorcluster, "Queue out"=w3782:refnum<queue>)  [unwired: 6 in]
        }
        n1614 = Initialize Array(FALSE ("element"), 6 ("dimension size")) -> (w3717:bool[])
        n1615 = Initialize Array(TRUE, 1 ("dimension size")) -> (w3716:bool[])
        n1616 = Merge Errors(w3752) -> (w3751:errorcluster)
        n1617 = Replace Array Subset(array=w3717, new element=w3716) -> (w3715:bool[])  [unwired: 1 in]
        n1618 = To Variant(anything=T3."mux10_1_channel6" ("mux10_1(x6)_encode")) -> (Variant=w3732:variant)
        n1619 = To Variant(anything=T4."demux1_10_channel6" ("demux1_10(x6)_encode")) -> (Variant=w3728:variant)
        n1620 = To Variant(anything=w3715) -> (Variant=w3724:variant)
        n1621 = Bundle By Name(cluster=w3721, "command"="MEAS.mux10-1", "data"=w3732) -> (w3727:T9)
        n1622 = Bundle By Name(cluster=w3721, "command"="MEAS.demux1-10", "data"=w3728) -> (w3726:T9)
        n1623 = Bundle By Name(cluster=w3721, "command"="MEAS.eMIC", "data"=w3724) -> (w3723:T9)
        n1624 = Build Array(w3727, w3726, w3723) -> (w3750:T9[])
        n1625 = Reverse 1D Array(array=w3750) -> (reversed array=w3749:T9[])
        n1626 = for {
          tunnel: w3749 -> [w3795] mode=indexing
          tunnel: [w3792] -> w3757 mode=indexing
          tunnel: w3751 -> [w3791]
          tunnel: w3754 -> [w3796]
          n1627 = Unbundle By Name(w3795) -> ("command"=w3794:string, "data"=w3793:variant)
          n1628 = call "App enquece.vi"("Priority Enquece"=TRUE, "error in (no error)"=w3791, "command data"=w3793, "command"=w3794, "queue in"=w3796) -> ("error out"=w3792:errorcluster)  [unwired: 5 in, 1 out]
        }
        n1629 = Merge Errors(w3760, w3757) -> (w3761:errorcluster)
      }
      frame "Test Channel 7A" {
        w3803 = T9 {"command"="", "data"=variant} ("element")
        w3824 = T9 {"command"="", "data"=variant} ("element")
        w3845 = 7  # DUT channel (1-10)
        n1630 = disable-structure shown="LOGGING==TRUE" {
          disable-tunnel: w3840 -> [w3869 _]
          frame condition #0 (active) {
            n1631 = Empty String/Path?(string/path=w3869) -> (empty?=w3871:bool)
            n1632 = Select(t="Quece timeout", s=w3871, f=w3869) -> (s? t:f=w3868:string)
            n1633 = call "string log (SubVI).vi"("state Name"=w3868) -> ()  [unwired: 9 in, 2 out]
          }
          frame condition #1 {
          }
        }
        n1634 = Bundle By Name(cluster=w3824, "command"="Apps.UI Update", "data"="A") -> (w3823:T9)
        n1635 = Bundle By Name(cluster=w3824, "command"="MEAS.AllRelaysOFF2") -> (w3822:T9)
        n1636 = Bundle By Name(cluster=w3824, "command"="Apps.WaitForEvent") -> (w3821:T9)
        n1637 = Build Array(w3823, w3822, w3821) -> (w3829:T9[])
        n1638 = call "FGV DRV stand.vi"() -> ("Sub-Test.DCV"=w3817:bool)  [unwired: 10 in, 1 out]
        n1639 = for {
          tunnel: [w3859] -> w3835 mode=indexing
          shift-right: [w3860] -> w3837
          shift-left: w3830 -> [w3858]
          tunnel: w3829 -> [w3857] mode=indexing
          n1640 = Unbundle By Name(w3857) -> ("command"=w3856:string, "data"=w3855:variant)
          n1641 = call "App enquece.vi"("Priority Enquece"=TRUE, "command data"=w3855, "command"=w3856, "queue in"=w3858) -> ("error out"=w3859:errorcluster, "Queue out"=w3860:refnum<queue>)  [unwired: 6 in]
        }
        n1642 = case shown="False" w3817 {
          tunnel: [w3848 w3854] -> w3838
          frame False {
            n1643 = Build Array("WaitFor", "MEAS.requestAC") -> (w3848:string[])
          }
          frame True {
            n1644 = Build Array("Test DRV 37", "WaitForA", "MEAS.requestAC") -> (w3854:string[])
          }
        }
        n1645 = Merge Errors(w3835) -> (w3828:errorcluster)
        n1646 = Reverse 1D Array(array=w3838) -> (reversed array=w3816:string[])
        n1647 = for {
          tunnel: w3816 -> [w3866] mode=indexing
          tunnel: [w3865] -> w3834 mode=indexing
          shift-right: [w3864] -> w3836
          shift-left: w3837 -> [w3867]
          tunnel: w3828 -> [w3863]
          n1648 = call "App enquece.vi"("Priority Enquece"=TRUE, "error in (no error)"=w3863, "command"=w3866, "queue in"=w3867) -> ("error out"=w3865:errorcluster, "Queue out"=w3864:refnum<queue>)  [unwired: 6 in]
        }
        n1649 = Merge Errors(w3834) -> (w3833:errorcluster)
        n1650 = Initialize Array(FALSE ("element"), 6 ("dimension size")) -> (w3799:bool[])
        n1651 = Initialize Array(TRUE, 1 ("dimension size")) -> (w3798:bool[])
        n1652 = Replace Array Subset(array=w3799, new element=w3798) -> (w3797:bool[])  [unwired: 1 in]
        n1653 = To Variant(anything=T3."mux10_1_channel7" ("mux10_1(x6)_encode")) -> (Variant=w3814:variant)
        n1654 = To Variant(anything=T4."demux1_10_channel7" ("demux1_10(x6)_encode")) -> (Variant=w3810:variant)
        n1655 = To Variant(anything=w3797) -> (Variant=w3806:variant)
        n1656 = Bundle By Name(cluster=w3803, "command"="MEAS.mux10-1", "data"=w3814) -> (w3809:T9)
        n1657 = Bundle By Name(cluster=w3803, "command"="MEAS.demux1-10", "data"=w3810) -> (w3808:T9)
        n1658 = Bundle By Name(cluster=w3803, "command"="MEAS.eMIC", "data"=w3806) -> (w3805:T9)
        n1659 = Build Array(w3809, w3808, w3805) -> (w3832:T9[])
        n1660 = Reverse 1D Array(array=w3832) -> (reversed array=w3831:T9[])
        n1661 = for {
          tunnel: w3831 -> [w3877] mode=indexing
          tunnel: [w3874] -> w3839 mode=indexing
          tunnel: w3833 -> [w3873]
          tunnel: w3836 -> [w3878]
          n1662 = Unbundle By Name(w3877) -> ("command"=w3876:string, "data"=w3875:variant)
          n1663 = call "App enquece.vi"("Priority Enquece"=TRUE, "error in (no error)"=w3873, "command data"=w3875, "command"=w3876, "queue in"=w3878) -> ("error out"=w3874:errorcluster)  [unwired: 5 in, 1 out]
        }
        n1664 = Merge Errors(w3842, w3839) -> (w3843:errorcluster)
      }
      frame "Test Channel 8A" {
        w3885 = T9 {"command"="", "data"=variant} ("element")
        w3906 = T9 {"command"="", "data"=variant} ("element")
        w3927 = 8  # DUT channel (1-10)
        n1665 = disable-structure shown="LOGGING==TRUE" {
          disable-tunnel: w3922 -> [w3951 _]
          frame condition #0 (active) {
            n1666 = Empty String/Path?(string/path=w3951) -> (empty?=w3953:bool)
            n1667 = Select(t="Quece timeout", s=w3953, f=w3951) -> (s? t:f=w3950:string)
            n1668 = call "string log (SubVI).vi"("state Name"=w3950) -> ()  [unwired: 9 in, 2 out]
          }
          frame condition #1 {
          }
        }
        n1669 = Bundle By Name(cluster=w3906, "command"="Apps.UI Update", "data"="A") -> (w3905:T9)
        n1670 = Bundle By Name(cluster=w3906, "command"="MEAS.AllRelaysOFF2") -> (w3904:T9)
        n1671 = Bundle By Name(cluster=w3906, "command"="Apps.WaitForEvent") -> (w3903:T9)
        n1672 = Build Array(w3905, w3904, w3903) -> (w3911:T9[])
        n1673 = for {
          tunnel: [w3941] -> w3917 mode=indexing
          shift-right: [w3942] -> w3919
          shift-left: w3912 -> [w3940]
          tunnel: w3911 -> [w3939] mode=indexing
          n1674 = Unbundle By Name(w3939) -> ("command"=w3938:string, "data"=w3937:variant)
          n1675 = call "App enquece.vi"("Priority Enquece"=TRUE, "command data"=w3937, "command"=w3938, "queue in"=w3940) -> ("error out"=w3941:errorcluster, "Queue out"=w3942:refnum<queue>)  [unwired: 6 in]
        }
        n1676 = call "FGV DRV stand.vi"() -> ("Sub-Test.DCV"=w3899:bool)  [unwired: 10 in, 1 out]
        n1677 = case shown="True" w3899 {
          tunnel: [w3930 w3936] -> w3920
          frame False {
            n1678 = Build Array("WaitFor", "MEAS.requestAC") -> (w3930:string[])
          }
          frame True {
            n1679 = Build Array("Test DRV 43", "WaitForA", "MEAS.requestAC") -> (w3936:string[])
          }
        }
        n1680 = Merge Errors(w3917) -> (w3910:errorcluster)
        n1681 = Reverse 1D Array(array=w3920) -> (reversed array=w3898:string[])
        n1682 = for {
          tunnel: w3898 -> [w3948] mode=indexing
          tunnel: [w3947] -> w3916 mode=indexing
          shift-right: [w3946] -> w3918
          shift-left: w3919 -> [w3949]
          tunnel: w3910 -> [w3945]
          n1683 = call "App enquece.vi"("Priority Enquece"=TRUE, "error in (no error)"=w3945, "command"=w3948, "queue in"=w3949) -> ("error out"=w3947:errorcluster, "Queue out"=w3946:refnum<queue>)  [unwired: 6 in]
        }
        n1684 = Initialize Array(FALSE ("element"), 6 ("dimension size")) -> (w3881:bool[])
        n1685 = Initialize Array(TRUE, 1 ("dimension size")) -> (w3880:bool[])
        n1686 = Merge Errors(w3916) -> (w3915:errorcluster)
        n1687 = Replace Array Subset(array=w3881, new element=w3880) -> (w3879:bool[])  [unwired: 1 in]
        n1688 = To Variant(anything=T3."mux10_1_channel8" ("mux10_1(x6)_encode")) -> (Variant=w3896:variant)
        n1689 = To Variant(anything=T4."demux1_10_channel8" ("demux1_10(x6)_encode")) -> (Variant=w3892:variant)
        n1690 = To Variant(anything=w3879) -> (Variant=w3888:variant)
        n1691 = Bundle By Name(cluster=w3885, "command"="MEAS.mux10-1", "data"=w3896) -> (w3891:T9)
        n1692 = Bundle By Name(cluster=w3885, "command"="MEAS.demux1-10", "data"=w3892) -> (w3890:T9)
        n1693 = Bundle By Name(cluster=w3885, "command"="MEAS.eMIC", "data"=w3888) -> (w3887:T9)
        n1694 = Build Array(w3891, w3890, w3887) -> (w3914:T9[])
        n1695 = Reverse 1D Array(array=w3914) -> (reversed array=w3913:T9[])
        n1696 = for {
          tunnel: w3913 -> [w3959] mode=indexing
          tunnel: [w3956] -> w3921 mode=indexing
          tunnel: w3915 -> [w3955]
          tunnel: w3918 -> [w3960]
          n1697 = Unbundle By Name(w3959) -> ("command"=w3958:string, "data"=w3957:variant)
          n1698 = call "App enquece.vi"("Priority Enquece"=TRUE, "error in (no error)"=w3955, "command data"=w3957, "command"=w3958, "queue in"=w3960) -> ("error out"=w3956:errorcluster)  [unwired: 5 in, 1 out]
        }
